vi "SQL_users_insert.vi"(9 "权限":i32, 10 "密码":string, 11 "用户名":string) -> (3 "error out":errorcluster)   [LabVIEW 2014]
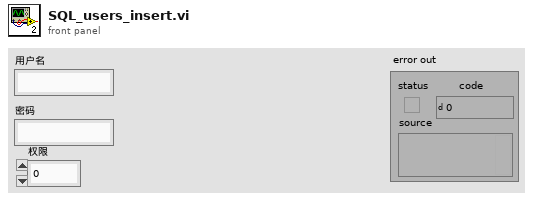
[diagram p1: front panel]
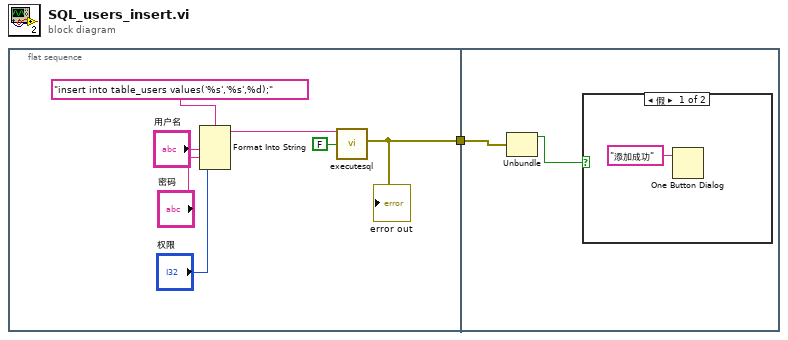
[diagram p0: block diagram]
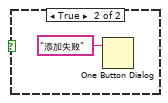
[diagram p2: hidden frame]
diagram:
  n1 = flat-sequence {
    tunnel: [w2] -> w1
    tunnel: w1 -> [w10]
    frame #0 {
      n2 = Format Into String(format string="insert into table_users values('%s','%s',%d);" ("Command Text"), "用户名", "密码", "权限") -> (resulting string=w7:string)  [unwired: 2 in, 1 out]
      n3 = call "executesql.vi"("Return Data (T)"=FALSE, "Command Text"=w7) -> ("error out"=w2:errorcluster)  [unwired: 5 in, 1 out]
      "error out" <- w2
    }
    frame #1 {
      n4 = Unbundle(w10) -> ("status"=w9:bool)  [unwired: 2 out]
      n5 = case shown="假" w9 {
        frame False {
          n6 = One Button Dialog(message="添加成功" ("消息")) -> ()  [unwired: 1 in, 1 out]
        }
        frame True {
          n7 = One Button Dialog(message="添加失败" ("消息")) -> ()  [unwired: 1 in, 1 out]
        }
      }
    }
  }
